vi "CreateSession.vi"(7 "DLL path":path, 8 "error in (no error)":errorcluster, 11 "ONNX model path":path) -> (0 "error out":errorcluster, 3 "session id out":i32)   [LabVIEW 2017, in "ONNX Class Library.lvlib"]
doc: "* @brief Создать новую сессию и загрузить ONNX модель в память\n * \n * Эта функция выделяет уникальный SessionID, загружает модель из файла,\n * анализирует её структуру (входы, выходы, типы данных, формы тензоров)\n * и сохраняет всю информацию для последующего использования.\n * \n * @param modelPath [IN] Путь к файлу модели в формате .onnx (абсолютный или относительный)\n * \n * @return int32: SessionID (положительное целое число >= 1) при успехе\n * @return int32: -1 при ошибке (неверный путь, повреждённая модель, нехватка памяти)\n * \n * @note SessionID необходимо сохранить и передавать во все последующие функции\n * @note При ошибке сессия автоматически удаляется из внутреннего хранилища\n */\nint CreateSession(const char* modelPath);"
uses:
  ONNX Class Library.lvlib
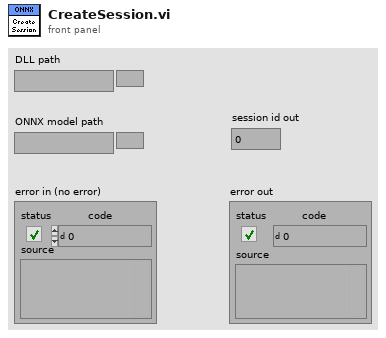
[diagram p1: front panel]
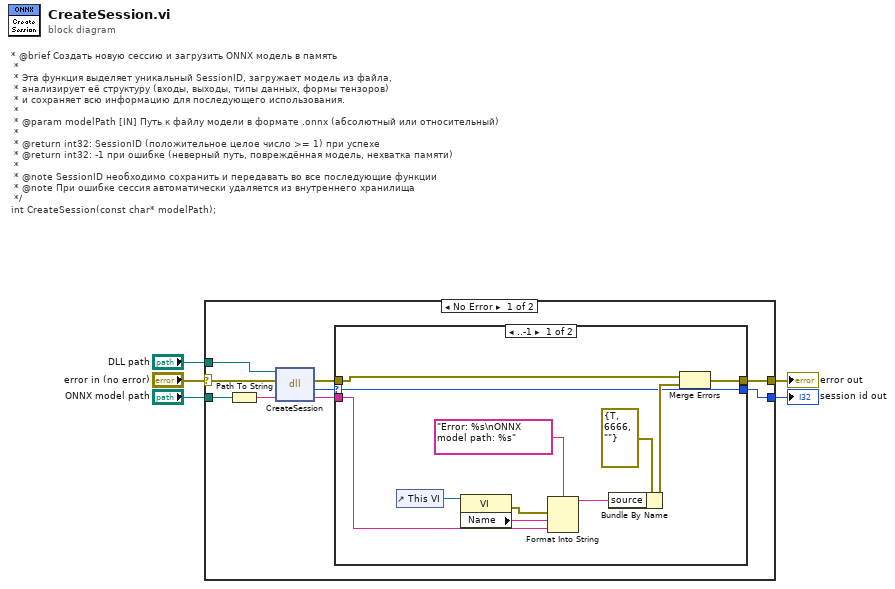
[diagram p0: block diagram]
diagram:
  # "* @brief Создать новую сессию и загрузить ONNX модель в память\n * \n * Эта функция выделяет уникальный SessionID, загружает модель из файла,\n * анализирует её структуру (входы, выходы, типы данных, формы тензоров)\n * и сохраняет всю информацию для последующего использования.\n * \n * @param modelPath [IN] Путь к файлу модели в формате .onnx (абсолютный или относительный)\n * \n * @return int32: SessionID (положительное целое число >= 1) при успехе\n * @return int32: -1 при ошибке (неверный путь, повреждённая модель, нехватка памяти)\n * \n * @note SessionID необходимо сохранить и передавать во все последующие функции\n * @note При ошибке сессия автоматически удаляется из внутреннего хранилища\n */\nint CreateSession(const char* modelPath);"
  n1 = case shown="No Error" "error in (no error)" {
    selector: "error in (no error)" -> [w7 w28]
    tunnel: "ONNX model path" -> [w14 _]
    tunnel: [w10 _] -> w4
    tunnel: [w9 w28] -> w3
    tunnel: "DLL path" -> [w6 _]
    frame No Error {
      n2 = Path To String(path=w14) -> (string=w13:string)
      n3 = dll-call lib="home/ivan/LabVIEWData/ONNX/Test/libonnx_wrapper/unix64/libonnx_wrapper.so" fn="CreateSession"(path in=w6, error in=w7, "modelPath"=w13) -> (error out=w12:errorcluster, "return"=w11:i32, "modelPath"=w8:string)  [unwired: 1 in, 1 out]
      n4 = case shown="..-1" w11 {
        selector: w11 -> [w15 w26]
        tunnel: w12 -> [w17 w27]
        tunnel: [w18 w27] -> w9
        tunnel: w8 -> [w16 _]
        tunnel: [w15 w26] -> w10
        frame ..-1 {
          n5 = control-ref of="This VI"() -> (w22:refnum<vi>)
          n6 = property class="VI"(reference=w22) -> (error out=w19:errorcluster, "Name"=w21:string)  [unwired: 1 in, 1 out]
          n7 = Format Into String(format string="Error: %s\nONNX model path: %s", error in=w19, w21, w16) -> (resulting string=w23:string)  [unwired: 1 in, 1 out]
          n8 = Bundle By Name(cluster=errorcluster {"status"=TRUE, "code"=6666, "source"=""} ("error out"), "source"=w23) -> (w24:errorcluster)
          n9 = Merge Errors(w17, w24) -> (w18:errorcluster)
        }
        frame 0.. {
        }
      }
    }
    frame Error {
    }
  }
  "session id out" <- w4
  "error out" <- w3
